vi "XNET TCP Socket Write (Binary).vi"(8 "error in":errorcluster, 9 "timeout ms (25000)":i32=25000, 10 "data":u8[](array[numeric]), 11 "socket in":refnum<k20>) -> (0 "error out":errorcluster, 2 "bytes written":i32, 3 "socket out":refnum<k20>)   [LabVIEW 2018]
doc: "Writes binary data to a TCP network connection."
uses:
  nixlvapi.dll
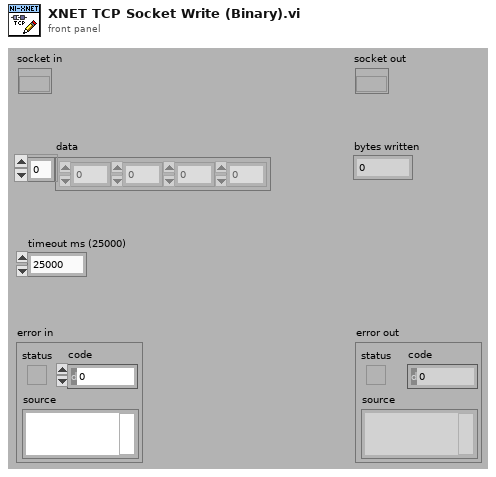
[diagram p1: front panel]
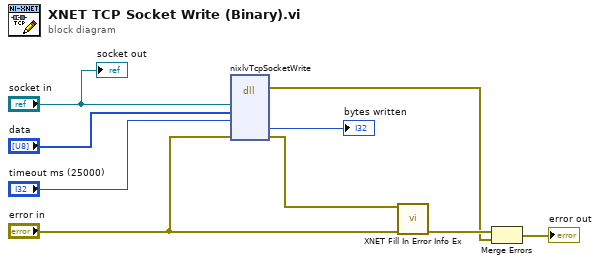
[diagram p0: block diagram]
diagram:
  n1 = dll-call lib="nixlvapi.*" fn="nixlvTcpSocketWrite" label="Call Library"("socketRef"="socket in", "lvData"="data", "timeoutMs"="timeout ms (25000)", "errorInOut"="error in") -> (error out=w7:errorcluster, "bytesWritten"=→"bytes written":i32, "errorInOut"=w9:errorcluster)  [unwired: 3 in, 6 out]
  n2 = call "XNET Fill In Error Info Ex.vi"("error xnet"=w9, "error in"="error in") -> ("error out"=w8:errorcluster)  [unwired: 13 in]
  n3 = Merge Errors(w8, w7) -> (→"error out":errorcluster)
  "socket out" <- "socket in"
